vi "get_js_from_tb.vi"(11 "lc_num":string) -> (0 "zc_luodi_num":string, 1 "jsren":string, 2 "jsbumen":string, 3 "zc_ini_state":string, 4 "error":errorcluster caption="error out 4", 6 "didian":string)   [LabVIEW 2017, in "Lib_code.lvlib"]
uses:
  Lib_code.lvlib
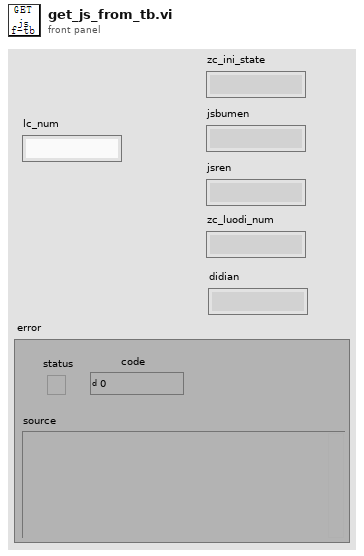
[diagram p1: front panel]
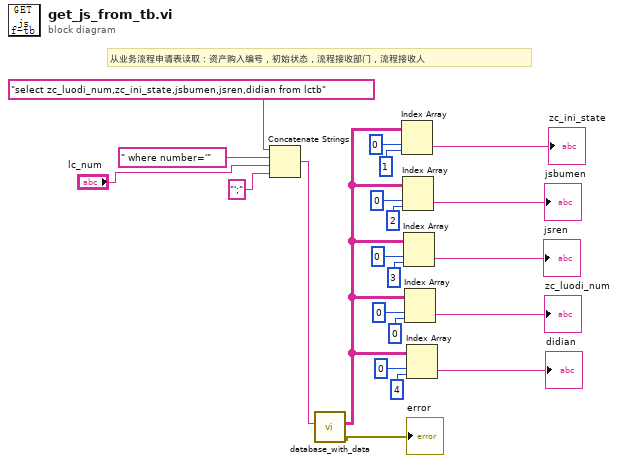
[diagram p0: block diagram]
diagram:
  # "从业务流程申请表读取：资产购入编号，初始状态，流程接收部门，流程接收人"
  n1 = Concatenate Strings("select zc_luodi_num,zc_ini_state,jsbumen,jsren,didian from lctb" ("Command Text"), " where number='" ("Command Text"), "lc_num", "';" ("字符串")) -> (w6:string)
  n2 = call "database_with_data.vi"("input"=w6) -> ("error"=→"error":errorcluster, "Data"=w2:string[][])  [unwired: 9 in]
  n3 = Index Array(array=w2, index (row)=0 ("索引 (行)"), index (col)=1 ("禁用的索引 (列)")) -> (element=→"zc_ini_state":string)
  n4 = Index Array(array=w2, index (row)=0 ("索引 (行)"), index (col)=2 ("禁用的索引 (列)")) -> (element=→"jsbumen":string)
  n5 = Index Array(array=w2, index (row)=0 ("索引 (行)"), index (col)=3 ("禁用的索引 (列)")) -> (element=→"jsren":string)
  n6 = Index Array(array=w2, index (row)=0 ("索引 (行)"), index (col)=0 ("禁用的索引 (列)")) -> (element=→"zc_luodi_num":string)
  n7 = Index Array(array=w2, index (row)=0 ("索引 (行)"), index (col)=4 ("禁用的索引 (列)")) -> (element=→"didian":string)
